vi "Integrate.vi"() -> (0 "Integral result":dbl)   [LabVIEW 2014]
panel:
  out "Array 2":i32[](array[numeric])
  out "Array":i32[](array[numeric])
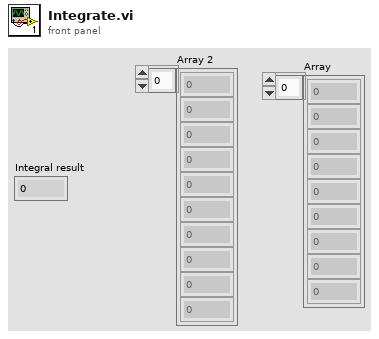
[diagram p1: front panel]
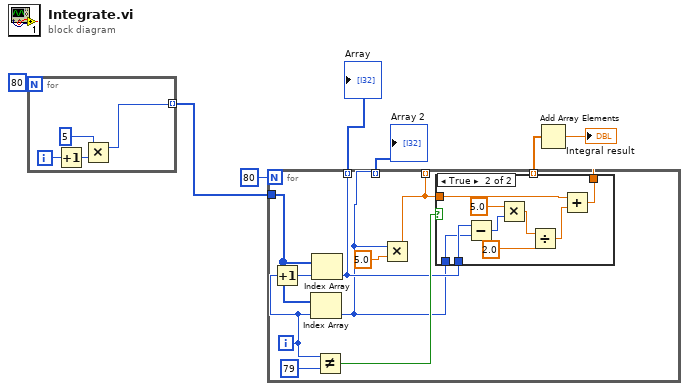
[diagram p0: block diagram]
diagram:
  n1 = for {
    N: 80 -> [_]
    tunnel: [w8] -> w3 mode=indexing
    i -> [w11]
    n2 = Increment(x=w11) -> (x+1=w10:i32)
    n3 = Multiply(x=5, y=w10) -> (x*y=w8:i32)
  }
  n4 = for {
    N: 80 -> [_]
    tunnel: [w21] -> w6 mode=indexing
    tunnel: w3 -> [w17]
    tunnel: [w14] -> _ mode=indexing
    tunnel: [w13] -> w2 mode=indexing
    tunnel: [w12] -> w1 mode=indexing
    i -> [w16]
    n5 = Increment(x=w16) -> (x+1=w15:i32)
    n6 = Index Array(array=w17, index=w16) -> (element=w12:i32)
    n7 = Index Array(array=w17, index=w15) -> (element=w13:i32)
    n8 = Not Equal?(x=w16, y=79) -> (x != y?=w18:bool)
    n9 = Multiply(x=w12, y=5.0) -> (x*y=w14:dbl)
    n10 = case shown="True" w18 {
      tunnel: w14 -> [w22 w27]
      tunnel: [w22 w26] -> w21
      tunnel: w13 -> [_ w25]
      tunnel: w12 -> [_ w24]
      frame False {
      }
      frame True {
        n11 = Subtract(x=w25, y=w24) -> (x-y=w31:i32)
        n12 = Multiply(x=5.0, y=w31) -> (x*y=w30:dbl)
        n13 = Divide(x=w30, y=2.0) -> (x/y=w28:dbl)
        n14 = Add(x=w27, y=w28) -> (x+y=w26:dbl)
      }
    }
  }
  "Array" <- w2
  "Array 2" <- w1
  n15 = Add Array Elements(numeric array=w6) -> (sum=→"Integral result":dbl)
